vi "Stop Core.vi"(10 "final error code":i32, 11 "Cylinder in":refnum<class "Cylinder.lvclass">) -> (3 "Cylinder out":refnum<class "Cylinder.lvclass">)   [LabVIEW 2015, in "cRIO-Carbondioxide.lvlib" / "CO2-Actor.lvlib" / "Cylinder.lvclass"]
doc: "(<B>Filename</B>: Actor Framework.lvlib:Actor.lvclass:Stop Core.vi)\n\nDefines what the actor does before it stops. Use the <B>final error code</B> input to determine whether the actor shut down in response to an error.\n\nBy default, this method does nothing. A descendant class may override it to define behavior, such as shutting down any processes the actor initiated in its override of the Actor Core method."
uses:
  Cylinder.lvclass
  Cylinder.lvclass/Cylinder.ctl
  <vilib>/ActorFramework/Message Enqueuer/Message Enqueuer.lvclass/Message Enqueuer.ctl
  <vilib>/ActorFramework/Message Enqueuer/Enqueue.vi
  <vilib>/ActorFramework/Message Priority Queue/Priority Enqueue.vi
  <vilib>/ActorFramework/Stop Msg/Stop Msg.lvclass
  CO2 Actor/CO2 Actor.lvclass
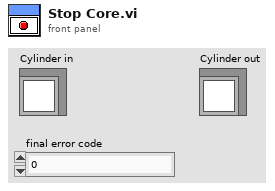
[diagram p1: front panel]
types:
  T1 = cluster{"Pressure Setpoint Control ":refnum<k21>, "Analog output":refnum<k21>, "Direction Valve IO":refnum<k21>, "Home Control":refnum<k21>, "Position Sensor":refnum<k21>}
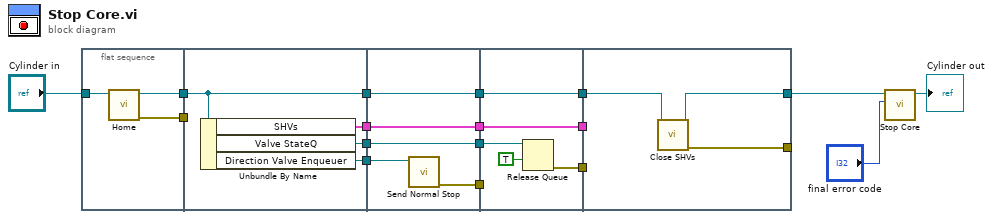
[diagram p0: block diagram]
diagram:
  n1 = flat-sequence {
    tunnel: "Cylinder in" -> [w20]
    tunnel: [w19] -> w13
    tunnel: [w18] -> w12
    tunnel: w13 -> [w24]
    tunnel: w12 -> [_]
    tunnel: [w24] -> w11
    tunnel: [w23] -> w10
    tunnel: [w22] -> w9
    tunnel: [w21] -> w8
    tunnel: w11 -> [w29]
    tunnel: w10 -> [w28]
    tunnel: w9 -> [w27]
    tunnel: w8 -> [w26]
    tunnel: [w29] -> w7
    tunnel: [w28] -> w6
    tunnel: [w27] -> w5
    tunnel: [w25] -> w4
    tunnel: w7 -> [w34]
    tunnel: w6 -> [w33]
    tunnel: w5 -> [w31]
    tunnel: w4 -> [_]
    tunnel: [w34] -> w3
    tunnel: [w33] -> w2
    tunnel: [w30] -> w1
    tunnel: [w36] -> w14
    tunnel: w3 -> [w37]
    tunnel: w2 -> [_]
    tunnel: w1 -> [_]
    tunnel: [w35] -> _
    frame #0 {
      n2 = call "Home.vi"("Cylinder in"=w20) -> ("error out"=w18:errorcluster, "Cylinder out"=w19:refnum<class "Cylinder.lvclass">)  [unwired: 9 in]
    }
    frame #1 {
      n3 = Unbundle By Name(w24) -> ("SHVs"=w23:T1, "Valve StateQ"=w22:refnum<queue>, "Direction Valve Enqueuer"=w21:refnum<class "Message Enqueuer.lvclass">)
    }
    frame #2 {
      n4 = call <vilib>:"Send Normal Stop.vi"("Message Enqueuer"=w26) -> ("error out"=w25:errorcluster)  [unwired: 10 in]
    }
    frame #3 {
      n5 = Release Queue(queue=w31, force destroy? (F)=TRUE) -> (error out=w30:errorcluster)  [unwired: 1 in, 2 out]
    }
    frame #4 {
      n6 = call "Close SHVs.vi"("Cylinder in"=w37) -> ("error out"=w35:errorcluster, "Cylinder out"=w36:refnum<class "Cylinder.lvclass">)  [unwired: 9 in]
    }
  }
  n7 = call-parent "Stop Core.vi"("final error code"="final error code", "CO2 Actor in"=w14) -> ("CO2 Actor out"=→"Cylinder out":refnum<class "Cylinder.lvclass">)  [unwired: 9 in]
